vi "Set IO Performance Graph Style.vi"(0 "Waveform Graph Refnum":refnum<vi>, 5 "# of plots (1)":i32=1, 7 "# of devices (1)":i32=1, 9 "Y maximum (1)":dbl[](array[numeric]), 11 "error in (no error)":errorcluster) -> (15 "error out":errorcluster)   [LabVIEW 2021]
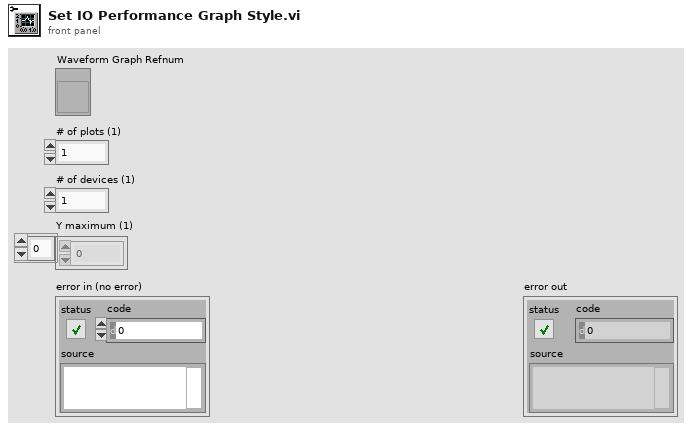
[diagram p1: front panel]
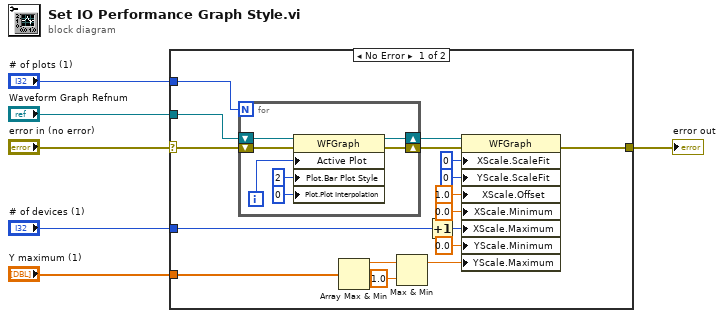
[diagram p0: block diagram]
diagram:
  n1 = case shown="No Error" "error in (no error)" {
    selector: "error in (no error)" -> [w18 w31]
    tunnel: "# of devices (1)" -> [w19 _]
    tunnel: "Waveform Graph Refnum" -> [w17 _]
    tunnel: "# of plots (1)" -> [w16 _]
    tunnel: "Y maximum (1)" -> [w10 _]
    tunnel: [w11 w31] -> w2
    frame No Error {
      n2 = for {
        N: w16 -> [_]
        shift-right: [w28] -> w13
        shift-left: w18 -> [w30]
        shift-right: [w24] -> w12
        shift-left: w17 -> [w29]
        i -> [w25]
        n3 = property class="WFGraph"(reference=w29, error in=w30, "Active Plot"=w25, "Plot.Bar Plot Style"=u8 2, "Plot.Plot Interpolation"=u8 0) -> (reference out=w24:refnum<vi>, error out=w28:errorcluster)
      }
      n4 = Array Max & Min(array=w10) -> (max value=w9:dbl)  [unwired: 3 out]
      n5 = Max & Min(x=w9, y=1.0) -> (max(x,y)=w7:dbl)  [unwired: 1 out]
      n6 = Increment(x=w19) -> (x+1=w21:i32)
      n7 = property class="WFGraph"(reference=w12, error in=w13, "XScale.ScaleFit"=u8 0 ("X Scale.Scale Fit"), "YScale.ScaleFit"=u8 0 ("Y Scale.Scale Fit"), "XScale.Offset"=1.0 ("X Scale.Offset and Multiplier:Offset"), "XScale.Minimum"=0.0 ("X Scale.Range:Minimum"), "XScale.Maximum"=w21, "YScale.Minimum"=0.0 ("Y Scale.Range:Minimum"), "YScale.Maximum"=w7) -> (error out=w11:errorcluster)  [unwired: 1 out]
    }
    frame Error {
    }
  }
  "error out" <- w2
